vi "LS_WRITE.vi"(8 "error in (no error)":errorcluster, 9 "write buffer":string, 10 "Data Cluster In":T3 {"GUI Data Cluster"."SBR" format="%08b"}, 11 "Config Cluster In":T1={"General"={"Config.ini"=path "", "Default Logging Path"=path ""}, "Hardware"={"Measure Rate (1/s)"=0, "HP DMM VISA"="", "LS 335 VISA"="", "HP DM"={"Range"=enum."Autorange", "Autozero"=FALSE, "Display"=enum."3 1/2 Digit", "Blank LCD"=FALSE}, "LS335"={"Brightness"=enum."25%"}}, "Operation"={"Operation Mode"=enum."Logging", "Status"="", "NewLog?"=FALSE, "OvenWarn"=FALSE, "LS335"={"Heater A"={"Range"=enum."Off", "Set Point"=0.0}, "Heater B"={"Range"=enum."Off", "Set Point"=0.0}}}}) -> (0 "error out":errorcluster, 1 "return count":u32, 2 "Data Cluster Out":T3 {"GUI Data Cluster"."SBR" format="%08b"}, 3 "Config Cluster Out":T1={"General"={"Config.ini"=path "", "Default Logging Path"=path ""}, "Hardware"={"Measure Rate (1/s)"=0, "HP DMM VISA"="", "LS 335 VISA"="", "HP DM"={"Range"=enum."Autorange", "Autozero"=FALSE, "Display"=enum."3 1/2 Digit", "Blank LCD"=FALSE}, "LS335"={"Brightness"=enum."25%"}}, "Operation"={"Operation Mode"=enum."Idle-Off", "Status"="", "NewLog?"=FALSE, "OvenWarn"=FALSE, "LS335"={"Heater A"={"Range"=enum."Off", "Set Point"=0.0}, "Heater B"={"Range"=enum."Off", "Set Point"=0.0}}}})   [LabVIEW 2021]
uses:
  Config_Cluster.ctl
  Mode_Enum.ctl
  Data_Cluster.ctl
  Measurement_Cluster.ctl
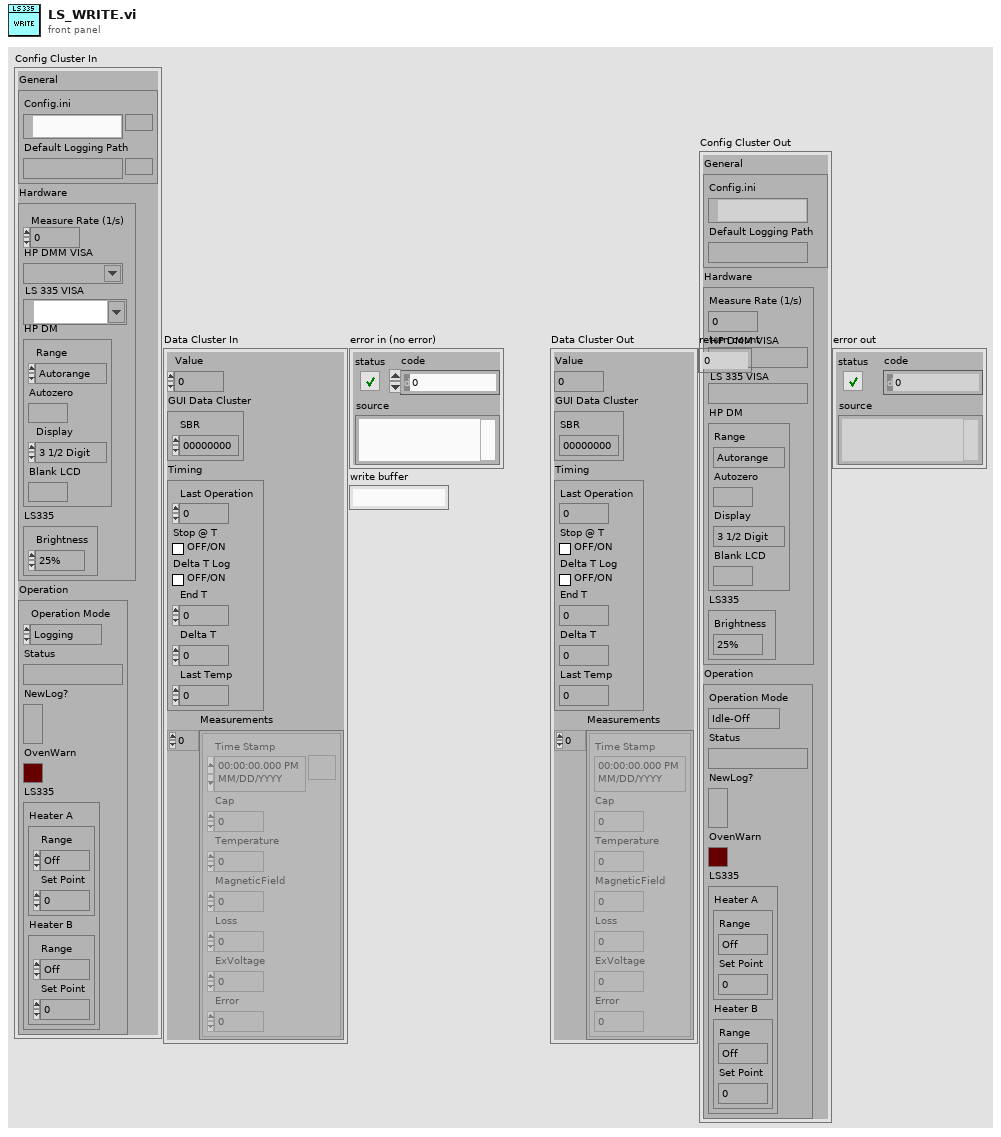
[diagram p1: front panel]
types:
  T1 = typedef "Config_Cluster.ctl" = cluster{"General":cluster{"Config.ini":path, "Default Logging Path":path}, "Hardware":cluster{"Measure Rate (1/s)":i32, "HP DMM VISA":refnum<visa-resource-name>, "LS 335 VISA":refnum<visa-resource-name>, "HP DM":cluster{"Range":enum16{"Autorange", "30mV", "300mV", "3V", "30V"}, "Autozero":bool, "Display":enum16{"3 1/2 Digit", "4 1/2 Digit", "5 1/2 Digit"}, "Blank LCD":bool}, "LS335":cluster{"Brightness":enum16{"25%", "50%", "75%", "100%"}}}, "Operation":cluster{"Operation Mode":T2, "Status":string, "NewLog?":bool, "OvenWarn":bool, "LS335":cluster{"Heater A":cluster{"Range":enum16{"Off", "Low", "Medium", "High"}, "Set Point":dbl}, "Heater B":cluster{"Range":enum16{"Off", "Low", "Medium", "High"}, "Set Point":dbl}}}}
  T2 = typedef "Mode_Enum.ctl" = enum16{"OvenNRDY", "Logging", "Idle-Off", "Idle"}
  T3 = typedef "Data_Cluster.ctl" = cluster{"Value":dbl, "GUI Data Cluster":cluster{"SBR":u16}, "Timing":cluster{"Last Operation":dbl, "Stop @ T":bool, "Delta T Log":bool, "End T":dbl, "Delta T":dbl, "Last Temp":dbl}, "Measurements":T4[]}
  T4 = typedef "Measurement_Cluster.ctl" = cluster{"Time Stamp":timestamp, "Cap":dbl, "Temperature":dbl, "MagneticField":dbl, "Loss":dbl, "ExVoltage":dbl, "Error":dbl}
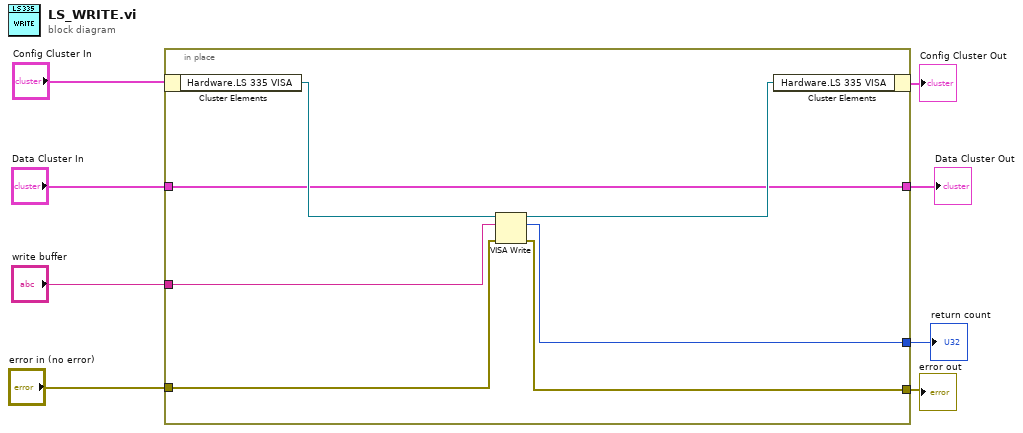
[diagram p0: block diagram]
diagram:
  n1 = in-place {
    in-place-border: "error in (no error)" -> [w13]
    in-place-border: [w12] -> w1
    in-place-border: "Data Cluster In" -> [w11]
    in-place-border: [w11] -> w5
    in-place-border: "write buffer" -> [w10]
    in-place-border: [w9] -> w2
    n2 = in-place-cluster #1("Config Cluster In") -> ("Hardware.LS 335 VISA"=w15:refnum<visa-resource-name>)
    n3 = VISA Write(VISA resource name=w15, write buffer=w10, error in (no error)=w13) -> (VISA resource name out=w14:refnum<visa-resource-name>, return count=w9:u32, error out=w12:errorcluster)
    n4 = in-place-cluster #1("Hardware.LS 335 VISA"=w14) -> (→"Config Cluster Out":T1)
  }
  "Data Cluster Out" <- w5
  "return count" <- w2
  "error out" <- w1
